vi "Change State.vi"(8 "error in (no error)":errorcluster, 10 "State":enum16{"INIT", "IDLE", "WORKING"}(ring), 11 "Chef Actor in":refnum<class "Chef Actor.lvclass">) -> (0 "error out":errorcluster, 3 "Chef Actor out":refnum<class "Chef Actor.lvclass">)   [LabVIEW 2024, in "Chef Actor.lvlib" / "Chef Actor.lvclass"]
uses:
  Chef Actor.lvclass
  Chef Actor.lvclass/Chef Actor.ctl
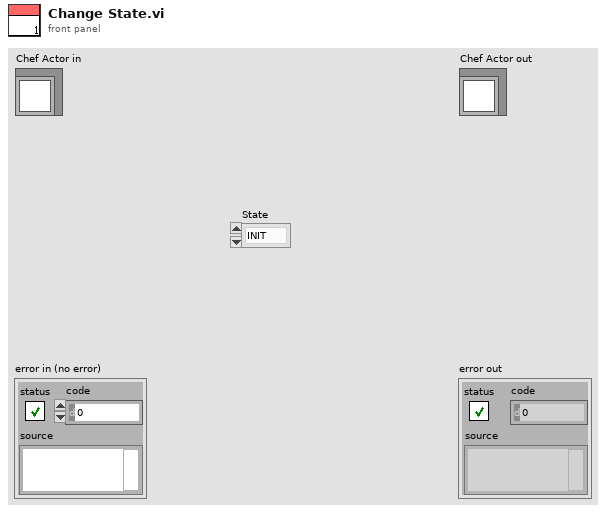
[diagram p1: front panel]
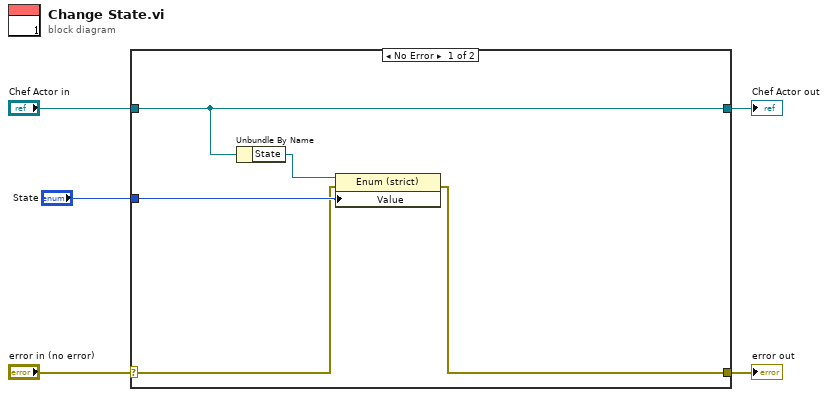
[diagram p0: block diagram]
diagram:
  n1 = case shown="No Error" "error in (no error)" {
    selector: "error in (no error)" -> [w7 w12]
    tunnel: [w6 w12] -> w4
    tunnel: [w10 w11] -> w2
    tunnel: "Chef Actor in" -> [w10 w11]
    tunnel: "State" -> [w8 _]
    frame No Error {
      n2 = Unbundle By Name(w10) -> ("State"=w9:refnum<vi>)
      n3 = property class="Enum (strict)"(reference=w9, error in=w7, "Value"=w8) -> (error out=w6:errorcluster)  [unwired: 1 out]
    }
    frame Error {
    }
  }
  "error out" <- w4
  "Chef Actor out" <- w2
